vi "GEA3 Read ERD (Rev 2 API).vi"(0 "GEA2 Reference In":refnum<k24>, 1 "Retry Count":i32=2 step=1, 2 "Read Timeout (ms)":u32=500, 5 "GEA Inputs":T4 {"Destination" format="%.0x"; "Source" format="%.0x"}, 7 "ERD Read Data In":T2 {"ERD Number" format="%.0x"}, 11 "Error In":errorcluster, 12 "Low Level Tries":u8=5 min=1, 13 "Verify ERD Response?":bool=TRUE) -> (4 "GEA2 Reference Out":refnum<k24>, 6 "Raw Data Out":string, 8 "ERD Read Data Out":T1 {"ERD Number" format="%.0x"}, 15 "Error Out":errorcluster)   [LabVIEW 2019, in "GEA2_Toolkit.lvlib"]
doc: "This VI reads an array of ERDs with a single command and returns the data in the data type selected."
uses:
  library/GEA2_Toolkit.lvlib
  C:/TechnologyLab/NI-2010/Drivers/GEA3 Toolkit/GEA3 DLL Source/GeaCommunication.dll
  GEA3 DLL Source/GeaCommunication.dll
  type defs/Source_Destination.ctl
  type defs/ERD Read Data In.ctl
  type defs/Data Type.ctl
  type defs/ERD Read Data Out.ctl
panel:
  out "Too Many Retries?":bool
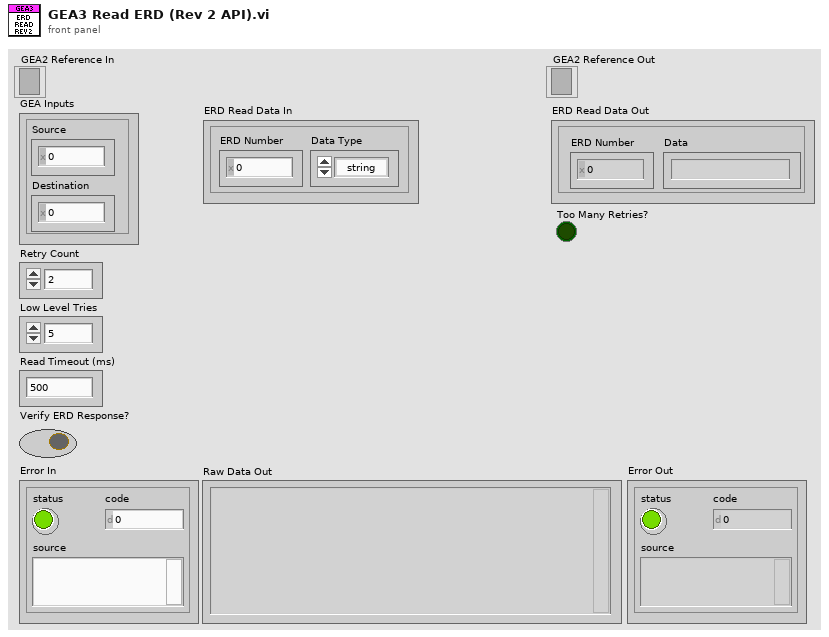
[diagram p1: front panel]
types:
  T1 = typedef "GEA2_Toolkit.lvlib/ERD Read Data Out.ctl" = cluster{"ERD Number":u16, "Data":string}
  T2 = typedef "GEA2_Toolkit.lvlib/ERD Read Data In.ctl" = cluster{"ERD Number":u16, "Data Type":T3}
  T3 = typedef "GEA2_Toolkit.lvlib/Data Type.ctl" = enum16{"string", "boolean", "uint8_t", "uint16_t", "uint32_t", "uint64_t", "int8_t", "int16_t", "int32_t", "int64_t"}
  T4 = typedef "GEA2_Toolkit.lvlib/Source_Destination.ctl" = cluster{"Source":u8, "Destination":u8}
  T5 = typedef "GEA2_Toolkit.lvlib/Data In.ctl" = cluster{"Source":u8, "Destination":u8, "Command":u8, "Message":string}
  T6 = typedef "GEA2_Toolkit.lvlib/Data Out.ctl" = cluster{"Source":u8, "Destination":u8, "Command":u8, "Length":u8, "CRC":u16, "Message":string}
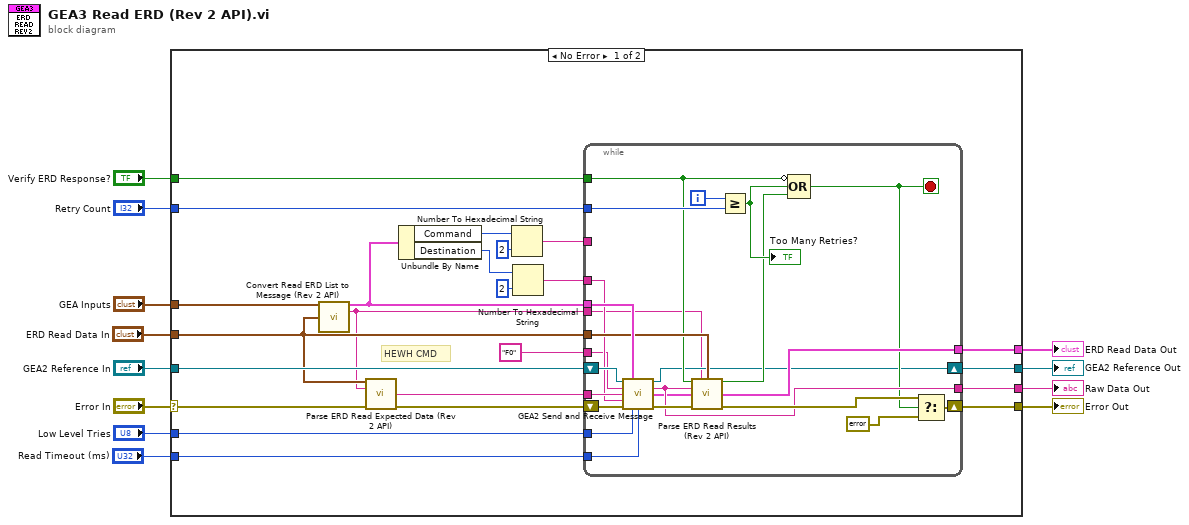
[diagram p0: block diagram]
diagram:
  n1 = case shown="No Error" "Error In" {
    selector: "Error In" -> [w35 w60]
    tunnel: "GEA2 Reference In" -> [w34 w61]
    tunnel: "ERD Read Data In" -> [w25 _]
    tunnel: "Verify ERD Response?" -> [w32 _]
    tunnel: "GEA Inputs" -> [w33 _]
    tunnel: [w28 _] -> w9
    tunnel: [w29 w60] -> w4
    tunnel: "Read Timeout (ms)" -> [w31 _]
    tunnel: "Retry Count" -> [w30 _]
    tunnel: [w27 w61] -> w6
    tunnel: [w26 _] -> w2
    tunnel: "Low Level Tries" -> [w24 _]
    frame No Error {
      # "HEWH CMD"
      n2 = call "Convert Read ERD List to Message (Rev 2 API).vi"("GEA Inputs"=w33, "ERD Read Data In"=w25) -> ("GEA Message"=w20:T5, "Request ID"=w13:string)  [unwired: 11 in, 1 out]
      n3 = call "Parse ERD Read Expected Data (Rev 2 API).vi"("ERD Read Data In"=w25, "Request ID"=w13, "Error In"=w35) -> ("Expected Data"=w23:string, "Error Out"=w22:errorcluster)  [unwired: 11 in]
      n4 = Unbundle By Name(w20) -> ("Command"=w19:u8, "Destination"=w16:u8)
      n5 = Number To Hexadecimal String(1:i16 2 ("width (-)"), 2:w19) -> (0:w18:string)
      n6 = Number To Hexadecimal String(1:i16 2 ("width (-)"), 2:w16) -> (0:w15:string)
      n7 = while {
        tunnel: w20 -> [w50]
        tunnel: [w43] -> w28
        tunnel: w32 -> [w41]
        tunnel: w25 -> [w44]
        tunnel: [w55] -> w26
        tunnel: w31 -> [w59]
        tunnel: w30 -> [w57]
        tunnel: w23 -> [w52]
        shift-right: [w45] -> w29
        shift-left: w22 -> [w51]
        shift-right: [w39] -> w27
        shift-left: w34 -> [w56]
        tunnel: w18 -> [_]
        tunnel: w24 -> [w49]
        tunnel: w15 -> [w38]
        tunnel: "F0" ("hex integer string") -> [w36]
        tunnel: w13 -> [w37]
        i -> [w58]
        stop <- w40 stop-if-true
        n8 = call "GEA2 Send and Receive Message.vi"("GEA2 Reference In"=w56, "Input Data"=w50, "Read Timeout (ms)"=w59, "Expected Command"=w36, "Expected Data"=w52, "Expected Source"=w38, "Error In"=w51, "# of Tries"=w49) -> ("GEA2 Reference Out"=w39:refnum<k24>, "Raw Data Out"=w43:string, "Converted Data Out"=w42:T6, "Error Out"=w48:errorcluster)  [unwired: 4 in]
        n9 = call "Parse ERD Read Results (Rev 2 API).vi"("Verify ERD Response?"=w41, "Request ID"=w37, "ERD Read Data In"=w44, "Raw Message"=w43, "Converted Data"=w42, "Error In"=w48) -> ("Pass/Fail?"=w53:bool, "ERD Read Data Out"=w55:T1, "Error Out"=w47:errorcluster)  [unwired: 7 in]
        n10 = Greater Or Equal?(x=w58, y=w57) -> (x >= y?=w54:bool)
        "Too Many Retries?" <- w54
        n11 = Compound Arithmetic op=OR(invert w41, w54, w53) -> (w40:bool)
        n12 = Select(t=w47, s=w40, f=errorcluster {"status"=FALSE, "code"=0, "source"=""}) -> (s? t:f=w45:errorcluster)
      }
    }
    frame Error {
    }
  }
  "Raw Data Out" <- w9
  "GEA2 Reference Out" <- w6
  "Error Out" <- w4
  "ERD Read Data Out" <- w2
